vi "A11rowmm.vi"(0 "Basic Size":dbl, 3 "error in (no error)":errorcluster) -> (5 "Row":i32, 8 "error out":errorcluster)   [LabVIEW 2023]
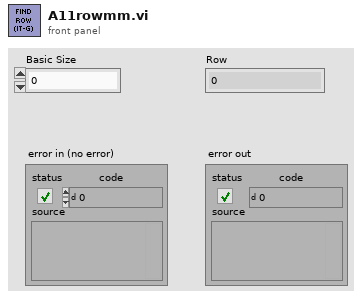
[diagram p1: front panel]
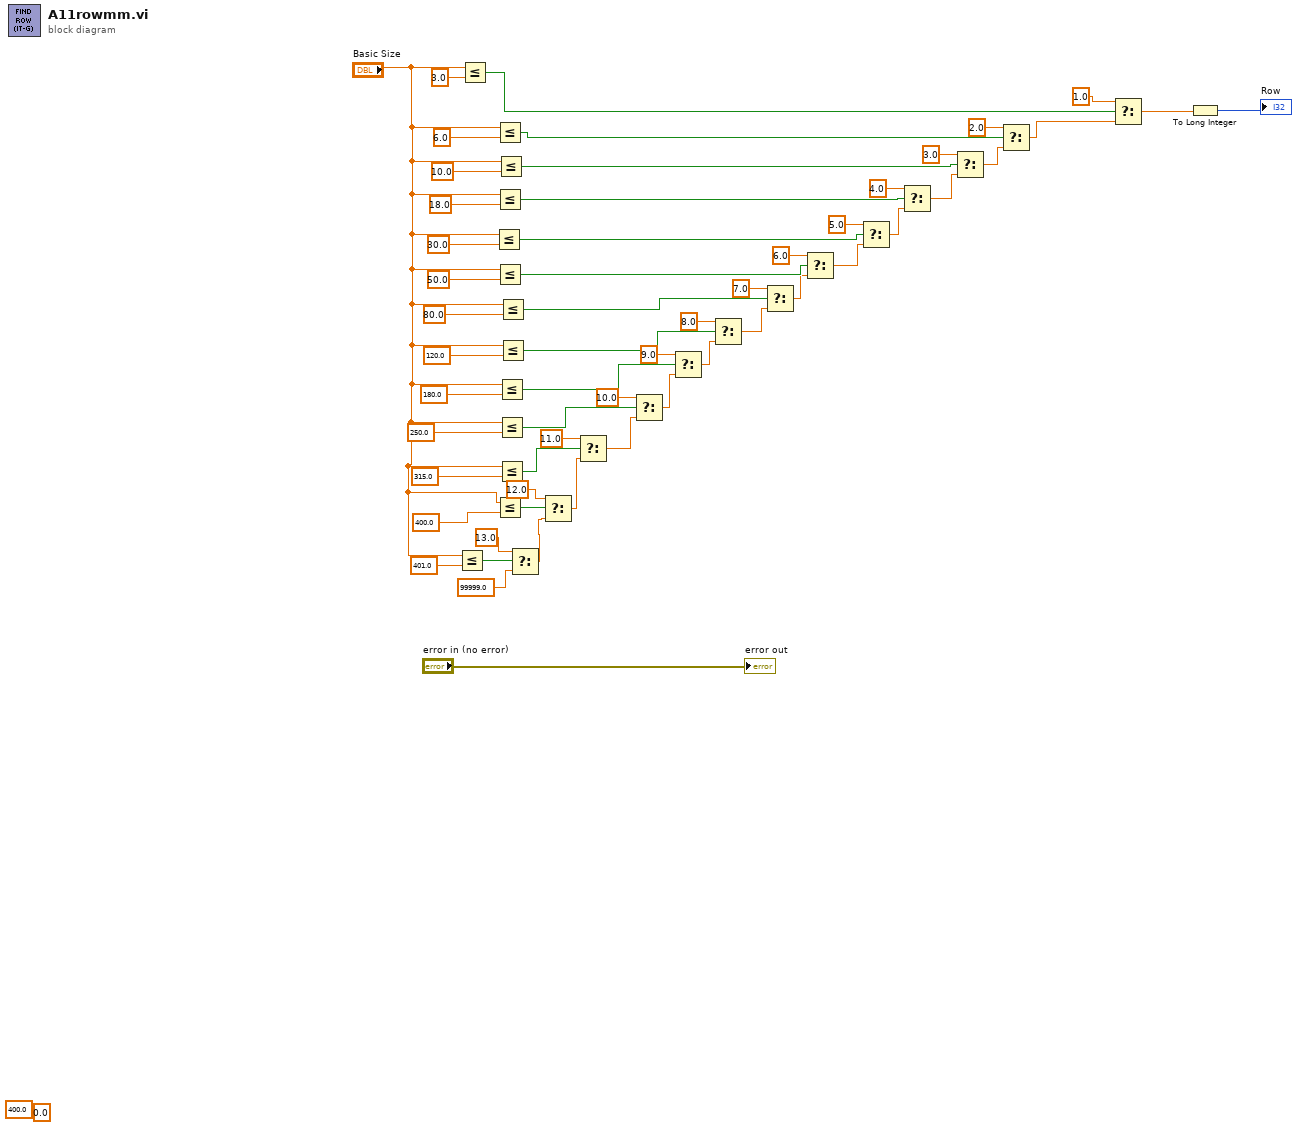
[diagram p0: block diagram]
diagram:
  (unwired) 0.0 ("f")
  (unwired) 400.0 ("y")
  n1 = Less Or Equal?(x="Basic Size", y=401.0) -> (x <= y?=w8:bool)
  n2 = Less Or Equal?(x="Basic Size", y=3.0) -> (x <= y?=w55:bool)
  n3 = Less Or Equal?(x="Basic Size", y=30.0) -> (x <= y?=w39:bool)
  n4 = Less Or Equal?(x="Basic Size", y=6.0) -> (x <= y?=w51:bool)
  n5 = Less Or Equal?(x="Basic Size", y=18.0) -> (x <= y?=w43:bool)
  n6 = Less Or Equal?(x="Basic Size", y=50.0) -> (x <= y?=w35:bool)
  n7 = Less Or Equal?(x="Basic Size", y=400.0 ("x")) -> (x <= y?=w13:bool)
  n8 = Less Or Equal?(x="Basic Size", y=10.0) -> (x <= y?=w48:bool)
  n9 = Less Or Equal?(x="Basic Size", y=180.0) -> (x <= y?=w23:bool)
  n10 = Less Or Equal?(x="Basic Size", y=250.0) -> (x <= y?=w19:bool)
  n11 = Less Or Equal?(x="Basic Size", y=315.0) -> (x <= y?=w15:bool)
  n12 = Less Or Equal?(x="Basic Size", y=80.0) -> (x <= y?=w31:bool)
  n13 = Less Or Equal?(x="Basic Size", y=120.0) -> (x <= y?=w27:bool)
  n14 = Select(t=13.0, s=w8, f=99999.0) -> (s? t:f=w7:dbl)
  n15 = Select(t=12.0, s=w13, f=w7) -> (s? t:f=w12:dbl)
  n16 = Select(t=11.0, s=w15, f=w12) -> (s? t:f=w17:dbl)
  n17 = Select(t=10.0, s=w19, f=w17) -> (s? t:f=w22:dbl)
  n18 = Select(t=9.0, s=w23, f=w22) -> (s? t:f=w25:dbl)
  n19 = Select(t=8.0, s=w27, f=w25) -> (s? t:f=w29:dbl)
  n20 = Select(t=7.0, s=w31, f=w29) -> (s? t:f=w33:dbl)
  n21 = Select(t=6.0, s=w35, f=w33) -> (s? t:f=w37:dbl)
  n22 = Select(t=5.0, s=w39, f=w37) -> (s? t:f=w41:dbl)
  n23 = Select(t=4.0, s=w43, f=w41) -> (s? t:f=w45:dbl)
  n24 = Select(t=3.0, s=w48, f=w45) -> (s? t:f=w49:dbl)
  n25 = Select(t=2.0, s=w51, f=w49) -> (s? t:f=w52:dbl)
  n26 = Select(t=1.0, s=w55, f=w52) -> (s? t:f=w9:dbl)
  n27 = To Long Integer(number=w9) -> (32bit integer=→"Row":i32)
  "error out" <- "error in (no error)"
